vi "onHttpPost (File).vi"(8 "error in":errorcluster, 10 "httpRequest":refnum<class "httpRequest.lvclass">, 11 "advanced-http-client in":refnum<class "advanced-http-client.lvclass">) -> (0 "error out":errorcluster, 2 "httpResponse":refnum<class "httpResponse.lvclass">, 3 "advanced-http-client out":refnum<class "advanced-http-client.lvclass">)   [LabVIEW 2020, in "HttpClient.NiAdvanced.lvlib" / "advanced-http-client.lvclass"]
uses:
  advanced-http-client.lvclass
  advanced-http-client.lvclass/advanced-http-client.ctl
  <vilib>/NI/Advanced HTTP Client/Session.lvclass
  http-client-pkg/httpRequest/httpRequest.lvclass
  <vilib>/NI/Advanced HTTP Client/POST (Buffer).vi
  http-client-pkg/httpResponse/httpResponse.lvclass
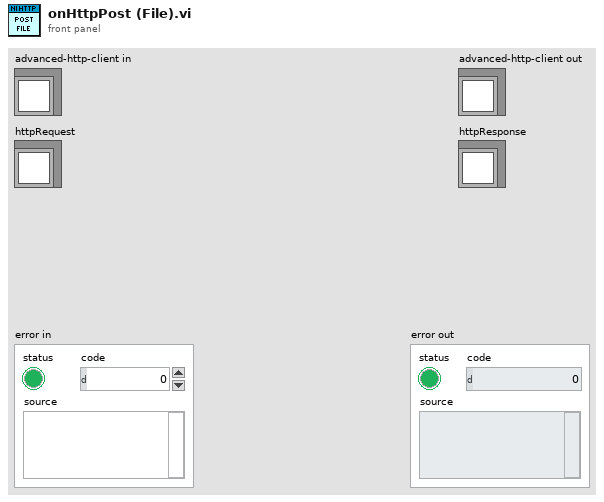
[diagram p1: front panel]
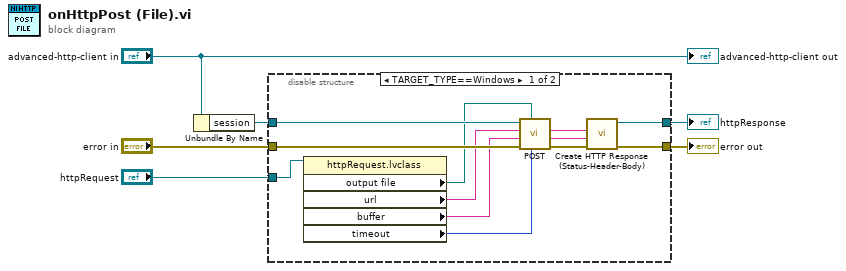
[diagram p0: block diagram]
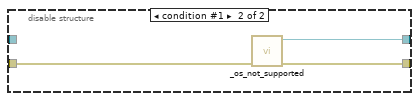
[diagram p2: hidden frame]
diagram:
  n1 = Unbundle By Name("advanced-http-client in") -> ("session"=w5:refnum<class "Session.lvclass">)
  n2 = disable-structure shown="TARGET_TYPE==Windows" {
    disable-tunnel: w5 -> [w18 _]
    disable-tunnel: "httpRequest" -> [w16 _]
    disable-tunnel: "error in" -> [w17 w21]
    disable-tunnel: [w7 w20] -> w2
    disable-tunnel: [w8 w19] -> w1
    frame condition #0 (active) {
      n3 = property class="httpRequest.lvclass"(reference=w16) -> ("output file"=w12:path, "url"=w15:string, "buffer"=w14:string, "timeout"=w13:i32)  [unwired: 1 in, 2 out]
      n4 = call-poly <vilib>:"POST.vi"("timeout"=w13, "output file"=w12, "error in"=w17, "buffer"=w14, "url"=w15, "session in"=w18) -> ("error out"=w11:errorcluster, "body"=w10:string, "headers"=w9:string)  [unwired: 1 in, 2 out]
      n5 = call "Create HTTP Response (Status-Header-Body).vi"("error in"=w11, "body"=w10, "Headers w/ status line(s)"=w9) -> ("error out"=w7:errorcluster, "httpResponse out"=w8:refnum<class "httpResponse.lvclass">)  [unwired: 7 in]
    }
    frame condition #1 {
      n6 = call "_os_not_supported.vi"("error in (no error)"=w21) -> ("error out"=w20:errorcluster, "httpResponse"=w19:refnum<class "httpResponse.lvclass">)  [unwired: 9 in]
    }
  }
  "error out" <- w2
  "httpResponse" <- w1
  "advanced-http-client out" <- "advanced-http-client in"
